vi "Init From Config.vi"(8 "error in (no error)":errorcluster, 10 "Carya Config in":refnum<class "Carya Config (By Reference).lvclass">, 11 "Carya Config in":refnum<class "Carya Config (By Reference).lvclass">) -> (0 "error out":errorcluster, 3 "Carya Config out":refnum<class "Carya Config (By Reference).lvclass">)   [LabVIEW 2013, in "Carya Config (By Reference).lvclass"]
doc: "Copyright 2018, Carya Automatisering, Wiebe Walstra."
uses:
  Carya Config (By Reference).lvclass
  Carya Config (By Reference).lvclass/Carya Config (By Reference).ctl
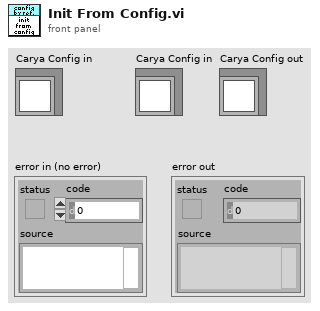
[diagram p1: front panel]
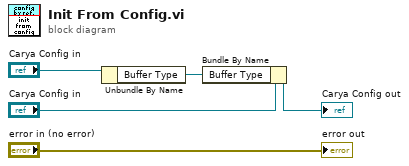
[diagram p0: block diagram]
diagram:
  n1 = Unbundle By Name("Carya Config in") -> ("Buffer Type"=w1:refnum<class "CConfig Buffer Type.lvclass">)
  n2 = Bundle By Name(cluster="Carya Config in", "Buffer Type"=w1) -> (→"Carya Config out":refnum<class "Carya Config (By Reference).lvclass">)
  "error out" <- "error in (no error)"
